vi "clear error.vi"(6 "wait for reply (T)":bool=TRUE, 8 "error in":errorcluster, 11 "Module ID":i32=-1) -> (0 "error out":errorcluster, 1 "timed out?":bool)   [LabVIEW 2025, in "Motor.lvlib"]
doc: "_____\nCreated using DQMH Framework: Event Scripter 7.1.2.1547."
uses:
  Motor.lvlib
  clear error Argument--cluster.ctl
  clear error (Reply Payload)--cluster.ctl
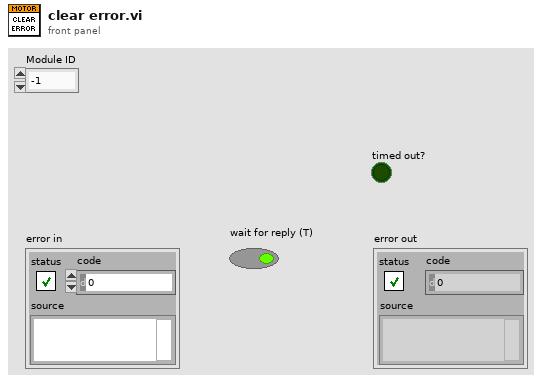
[diagram p1: front panel]
types:
  T1 = typedef "Motor.lvlib/clear error Argument--cluster.ctl" = cluster{"Module ID":i32, "Wait Notifier":refnum<notifier>, "wait for reply":bool}
  T2 = typedef "Motor.lvlib/Request Events--cluster.ctl" = cluster{"Stop Module":refnum<user-event>, "Show Panel":refnum<user-event>, "Hide Panel":refnum<user-event>, "Show Diagram":refnum<user-event>, "Get Module Execution Status":refnum<user-event>, "close":refnum<user-event>, "init":refnum<user-event>, "clear error":refnum<user-event>}
  T3 = typedef "Motor.lvlib/clear error (Reply Payload)--cluster.ctl" = cluster{"Module ID":i32, "error":errorcluster}
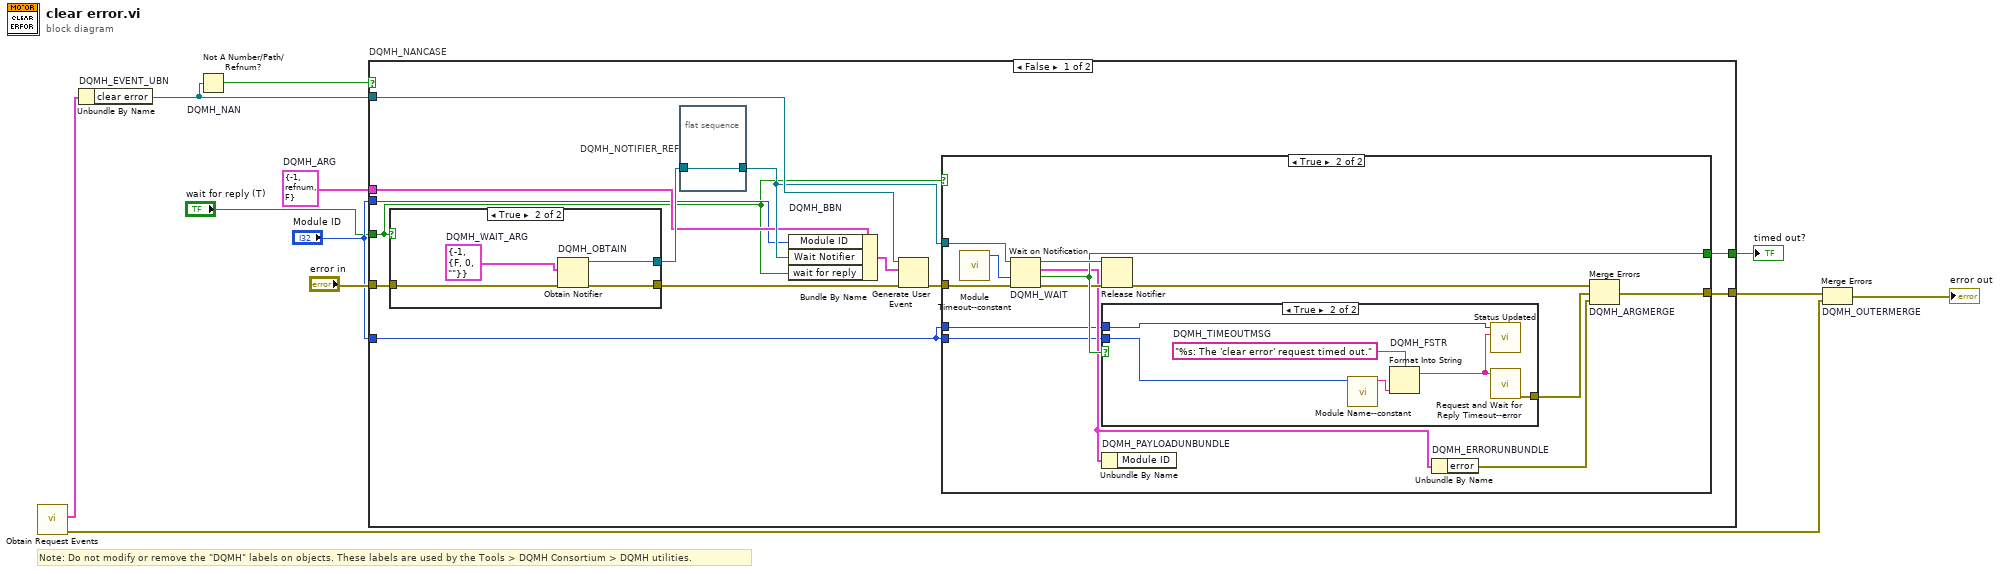
[diagram p0: block diagram]
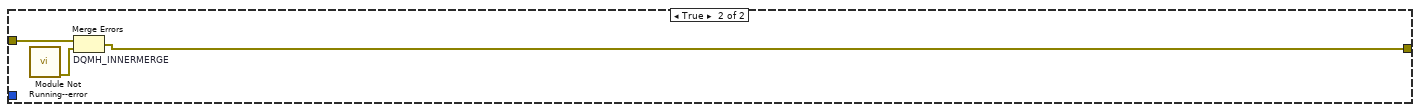
[diagram p5: hidden frame]
diagram:
  w5 = T1 {"Module ID"=-1, "Wait Notifier"=refnum, "wait for reply"=FALSE}  # DQMH_ARG
  # "Note: Do not modify or remove the \"DQMH\" labels on objects. These labels are used by the Tools > DQMH Consortium > DQMH utilities."
  n1 = call "Obtain Request Events.vi"() -> ("error out"=w2:errorcluster, "Motor Request Events"=w1:T2)  [unwired: 10 in]
  n2 = Unbundle By Name "DQMH_EVENT_UBN"(w1) -> ("clear error"=w9:refnum<user-event>)
  n3 = Not A Number/Path/Refnum? "DQMH_NAN"(number/path/refnum=w9) -> (NaN/Path/Refnum?=w8:bool)
  n4 = case "DQMH_NANCASE" shown="False" w8 {
    tunnel: "error in" -> [w24 w53]
    tunnel: w9 -> [w22 _]
    tunnel: [w19 w52] -> w6
    tunnel: [w20 _] -> w7
    tunnel: w5 -> [w15 _]
    tunnel: "Module ID" -> [w14 _]
    tunnel: "Module ID" -> [w13 _]
    tunnel: "wait for reply (T)" -> [w12 _]
    frame False {
      n5 = case shown="True" w12 {
        tunnel: w24 -> [w46 w50]
        tunnel: [w46 w49] -> w21
        tunnel: [_ w47] -> w17
        frame False {
        }
        frame True {
          w48 = T3 {"Module ID"=-1, "error"={"status"=FALSE, "code"=0, "source"=""}}  # DQMH_WAIT_ARG
          n6 = Obtain Notifier "DQMH_OBTAIN"(notification data type=w48, error in (no error)=w50) -> (notifier out=w47:refnum<notifier>, error out=w49:errorcluster)  [unwired: 2 in, 1 out]
        }
      }
      n7 = flat-sequence "DQMH_NOTIFIER_REF" {
        tunnel: w17 -> [w25]
        tunnel: [w25] -> w16
        frame #0 {
        }
      }
      n8 = Bundle By Name "DQMH_BBN"(cluster=w15, "Module ID"=w14, "Wait Notifier"=w16, "wait for reply"=w12) -> (w18:T1)
      n9 = Generate User Event(user event=w22, event data cluster=w18, error in=w21) -> (error out=w23:errorcluster)  [unwired: 1 in, 1 out]
      n10 = case shown="True" w12 {
        tunnel: w23 -> [w26 w39]
        tunnel: w16 -> [_ w38]
        tunnel: [_ w36] -> w20
        tunnel: [w26 w35] -> w19
        tunnel: w13 -> [_ w28]
        tunnel: w13 -> [_ w27]
        frame False {
        }
        frame True {
          n11 = call "Module Timeout--constant.vi"() -> ("Module Timeout"=w29:i32)  [unwired: 11 in]
          n12 = Wait on Notification "DQMH_WAIT"(notifier=w38, timeout in ms (-1)=w29, error in (no error)=w39) -> (notifier out=w37:refnum<notifier>, notification=w30:T3, timed out?=w36:bool, error out=w34:errorcluster)  [unwired: 1 in]
          n13 = Release Notifier(notifier=w37, error in (no error)=w34) -> (error out=w33:errorcluster)  [unwired: 1 in, 2 out]
          n14 = case shown="True" w36 {
            tunnel: [_ w43] -> w31
            tunnel: w28 -> [_ w41]
            tunnel: w27 -> [_ w40]
            frame False {
            }
            frame True {
              w45 = "%s: The 'clear error' request timed out."  # DQMH_TIMEOUTMSG
              n15 = call "Module Name--constant.vi"("Module ID"=w40) -> ("Module Name"=w42:string)  [unwired: 10 in]
              n16 = Format Into String "DQMH_FSTR"(format string=w45, w42) -> (resulting string=w44:string)  [unwired: 2 in, 1 out]
              n17 = call "Status Updated.vi"("Status"=w44, "Module ID"=w41) -> ()  [unwired: 9 in, 1 out]
              n18 = call "Request and Wait for Reply Timeout--error.vi"("Error Message"=w44) -> ("error out"=w43:errorcluster)  [unwired: 10 in]
            }
          }
          n19 = Unbundle By Name "DQMH_PAYLOADUNBUNDLE"(w30) -> ()  [unwired: 1 out]
          n20 = Unbundle By Name "DQMH_ERRORUNBUNDLE"(w30) -> ("error"=w32:errorcluster)
          n21 = Merge Errors "DQMH_ARGMERGE"(w33, w31, w32) -> (w35:errorcluster)
        }
      }
    }
    frame True {
      n22 = call "Module Not Running--error.vi"() -> ("error out"=w51:errorcluster)  [unwired: 11 in]
      n23 = Merge Errors "DQMH_INNERMERGE"(w53, w51) -> (w52:errorcluster)
    }
  }
  "timed out?" <- w7
  n24 = Merge Errors "DQMH_OUTERMERGE"(w6, w2) -> (→"error out":errorcluster)
